vi "SECoP_dataGetBlob.vi"(7 "Position":u32, 8 "error in (no error)":errorcluster, 10 "SECoP_dataPtr in":T1 {"ptr64" format="%.0x"; "ptr32" format="%.0x"}, 11 "DLL path (in)":T2) -> (0 "error out":errorcluster, 2 "Value":u8[](array[numeric]), 3 "DLL path (out)":T2)   [LabVIEW 2023, in "SECoP.lvlib"]
doc: "Call <b>\"SECoP_dataGetBlob.vi\"</b> to access the contained binary large object (BLOB of SECoP_dataPtr).\n\n<b>DLL path</b> input and output of cluster from \"SECoP-Initialize.vi\"\n<b>SECoP_dataPtr</b> data to access\n<b>Position</b> points to a virtual flattened entry of the data type\n<b>Value</b> byte array of BLOB"
uses:
  SECoP.lvlib
  SECoP-libraries.ctl
  SECoP-data.ctl
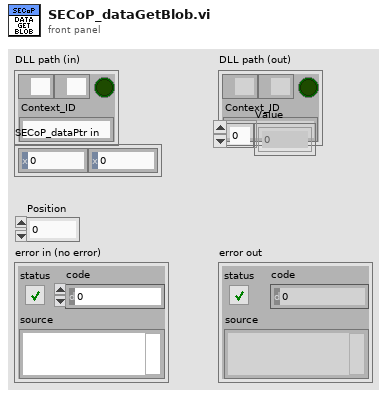
[diagram p1: front panel]
types:
  T1 = typedef "SECoP.lvlib/SECoP-data.ctl" = cluster{"ptr32":u32, "ptr64":u64}
  T2 = typedef "SECoP.lvlib/SECoP-libraries.ctl" = cluster{"serverDLL":path, "variantDLL":path, "cleanup_mode":bool, "Context_ID":string}
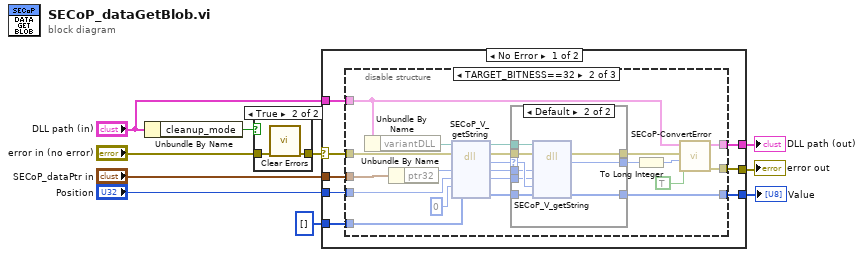
[diagram p0: block diagram]
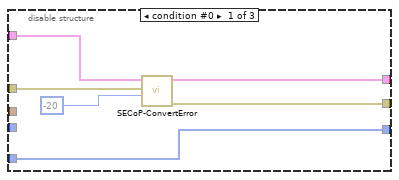
[diagram p2: hidden frame]
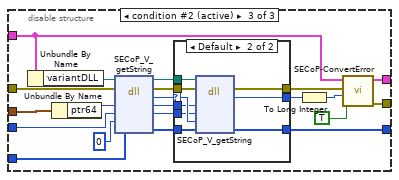
[diagram p4: hidden frame]
diagram:
  n1 = Unbundle By Name("DLL path (in)") -> ("cleanup_mode"=w7:bool)
  n2 = case shown="True" w7 {
    tunnel: "error in (no error)" -> [w11 w13]
    tunnel: [w11 w12] -> w5
    frame False {
    }
    frame True {
      n3 = call <vilib>:"Clear Errors.vi"("error in (no error)"=w13) -> ("error out"=w12:errorcluster)  [unwired: 5 in, 1 out]
    }
  }
  n4 = case shown="No Error" w5 {
    selector: w5 -> [w21 w95]
    tunnel: "DLL path (in)" -> [w20 w96]
    tunnel: [w16 w96] -> w9
    tunnel: [w17 w95] -> w8
    tunnel: "Position" -> [w19 _]
    tunnel: [w18 w94] -> w3
    tunnel: "SECoP_dataPtr in" -> [w15 _]
    tunnel: u8[] [] ("Value") -> [w14 w94]
    frame No Error {
      n5 = disable-structure shown="TARGET_BITNESS==32" {
        disable-tunnel: w21 -> [w25 w48 w81]
        disable-tunnel: w20 -> [w26 w28 w61]
        disable-tunnel: w19 -> [_ w47 w80]
        disable-tunnel: [w22 w30 w63] -> w18
        disable-tunnel: w14 -> [w22 w43 w76]
        disable-tunnel: [w24 w32 w65] -> w17
        disable-tunnel: [w27 w33 w66] -> w16
        disable-tunnel: w15 -> [_ w46 w79]
        frame condition #0 {
          n6 = call "SECoP-ConvertError.vi"("return code"=-20, "error in (no error)"=w25, "DLL path (in)"=w26) -> ("error out"=w24:errorcluster, "DLL path (out)"=w27:T2)  [unwired: 7 in]
        }
        frame condition #1 {
          n7 = Unbundle By Name(w28) -> ("variantDLL"=w29:path)
          n8 = Unbundle By Name(w46) -> ("ptr32"=w45:u32)
          n9 = dll-call lib="Z:/Praktische_Aufgaben/SECoP-LabVIEW2015/32bit/SECoP32.dll" fn="SECoP_V_getString"(path in=w29, error in=w48, "pData"=w45, "uPosition"=w47, "uBufferSize"=u32 0 ("BufferSize"), "pValue"=w43) -> (path out=w42:path, error out=w37:errorcluster, "return type"=w41:u32, "pData"=w40:u32, "uPosition"=w39:u32, "pValue"=w38:u8[])  [unwired: 2 in]
          n10 = case shown="Default" w41 {
            selector: w41 -> [w51 w59]
            tunnel: w42 -> [_ w60]
            tunnel: w40 -> [_ w58]
            tunnel: w39 -> [_ w57]
            tunnel: w38 -> [w49 w56]
            tunnel: [w49 w55] -> w30
            tunnel: w37 -> [w50 w54]
            tunnel: [w50 w53] -> w34
            tunnel: [w51 w52] -> w31
            frame 0 {
            }
            frame Default {
              n11 = dll-call lib="Z:/Praktische_Aufgaben/SECoP-LabVIEW2015/32bit/SECoP32.dll" fn="SECoP_V_getString"(path in=w60, error in=w54, "pData"=w58, "uPosition"=w57, "uBufferSize"=w59, "pValue"=w56) -> (error out=w53:errorcluster, "return type"=w52:u32, "pValue"=w55:u8[])  [unwired: 4 in, 1 out]
            }
          }
          n12 = To Long Integer(number=w31) -> (32bit integer=w36:i32)
          n13 = call "SECoP-ConvertError.vi"("return is boolean"=TRUE, "return code"=w36, "error in (no error)"=w34, "DLL path (in)"=w28) -> ("error out"=w32:errorcluster, "DLL path (out)"=w33:T2)  [unwired: 6 in]
        }
        frame condition #2 (active) {
          n14 = Unbundle By Name(w61) -> ("variantDLL"=w62:path)
          n15 = Unbundle By Name(w79) -> ("ptr64"=w78:u64)
          n16 = dll-call lib="Z:/Praktische_Aufgaben/SECoP-LabVIEW2015/32bit/SECoP32.dll" fn="SECoP_V_getString"(path in=w62, error in=w81, "pData"=w78, "uPosition"=w80, "uBufferSize"=u32 0 ("BufferSize"), "pValue"=w76) -> (path out=w75:path, error out=w70:errorcluster, "return type"=w74:u32, "pData"=w73:u64, "uPosition"=w72:u32, "pValue"=w71:u8[])  [unwired: 2 in]
          n17 = case shown="Default" w74 {
            selector: w74 -> [w84 w92]
            tunnel: w75 -> [_ w93]
            tunnel: w73 -> [_ w91]
            tunnel: w72 -> [_ w90]
            tunnel: w71 -> [w82 w89]
            tunnel: [w82 w88] -> w63
            tunnel: w70 -> [w83 w87]
            tunnel: [w83 w86] -> w67
            tunnel: [w84 w85] -> w64
            frame 0 {
            }
            frame Default {
              n18 = dll-call lib="Z:/Praktische_Aufgaben/SECoP-LabVIEW2015/32bit/SECoP32.dll" fn="SECoP_V_getString"(path in=w93, error in=w87, "pData"=w91, "uPosition"=w90, "uBufferSize"=w92, "pValue"=w89) -> (error out=w86:errorcluster, "return type"=w85:u32, "pValue"=w88:u8[])  [unwired: 4 in, 1 out]
            }
          }
          n19 = To Long Integer(number=w64) -> (32bit integer=w69:i32)
          n20 = call "SECoP-ConvertError.vi"("return is boolean"=TRUE, "return code"=w69, "error in (no error)"=w67, "DLL path (in)"=w61) -> ("error out"=w65:errorcluster, "DLL path (out)"=w66:T2)  [unwired: 6 in]
        }
      }
    }
    frame Error {
    }
  }
  "DLL path (out)" <- w9
  "error out" <- w8
  "Value" <- w3
